vi "calc_complex_to_abs_phase.vi"(7 "index":i32, 11 "complex value":dbl[](array[numeric])) -> (3 "output":cluster{"abs":dbl, "phase":dbl})   [LabVIEW 2025]
panel:
  out "phase":dbl
  out "abs":dbl
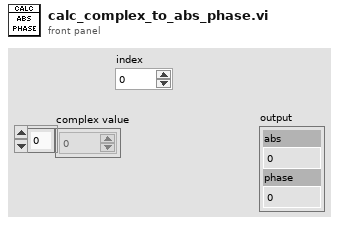
[diagram p1: front panel]
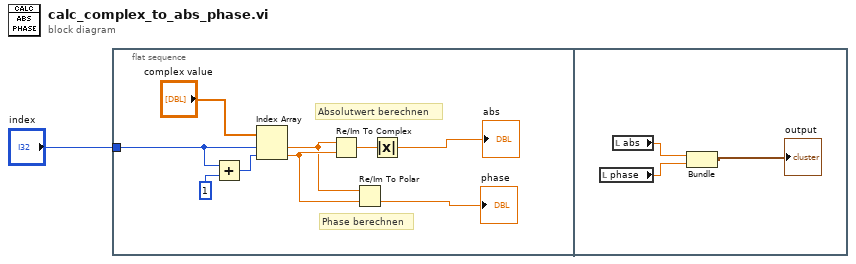
[diagram p0: block diagram]
diagram:
  n1 = flat-sequence {
    tunnel: "index" -> [w3]
    frame #0 {
      # "Phase berechnen"
      # "Absolutwert berechnen"
      n2 = Add(x=w3, y=1) -> (x+y=w4:i32)
      n3 = Index Array(array="complex value", index #1=w3, index #2=w4) -> (element #1=w7:dbl, element #2=w8:dbl)
      n4 = Re/Im To Complex(1:w8, 2:w7) -> (0:w6:cdb)
      n5 = Re/Im To Polar(2:w8, 3:w7) -> (0:→"phase":dbl)  [unwired: 1 out]
      n6 = Absolute Value(x=w6) -> (abs(x)=→"abs":dbl)
    }
    frame #1 {
      n7 = local read "phase"() -> (w12:dbl)
      n8 = local read "abs"() -> (w11:dbl)
      n9 = Bundle("abs"=w11, "phase"=w12) -> (→"output":cluster{"abs":dbl, "phase":dbl})  [unwired: 1 in]
    }
  }
